vi "PXI4072 Set Refs.vi"(8 "error in (no error)":errorcluster, 11 "PXI4072 All UI Refs":T1) -> (0 "error out":errorcluster)   [LabVIEW 2026]
uses:
  App Types/References/PXI4072 All UI References.ctl
  App Types/References/PXI4072 Boolean UI References.ctl
  App Types/References/PXI4072 String UI References.ctl
  App Types/References/PXI4072 Numeric UI References.ctl
  App Types/References/PXI4072 Other UI Rerences.ctl
  Drivers/PXI4072/Types/PXI4072 Settings.ctl
  <instrlib>/niDMM/nidmm.llb/niDMM Function.ctl
  <instrlib>/niDMM/nidmm.llb/niDMM Resolution in Digits.ctl
  App Types/Globals/PXI4072 UI Global Refs.vi
  Drivers/PXI4072/PXI4072.lvlib
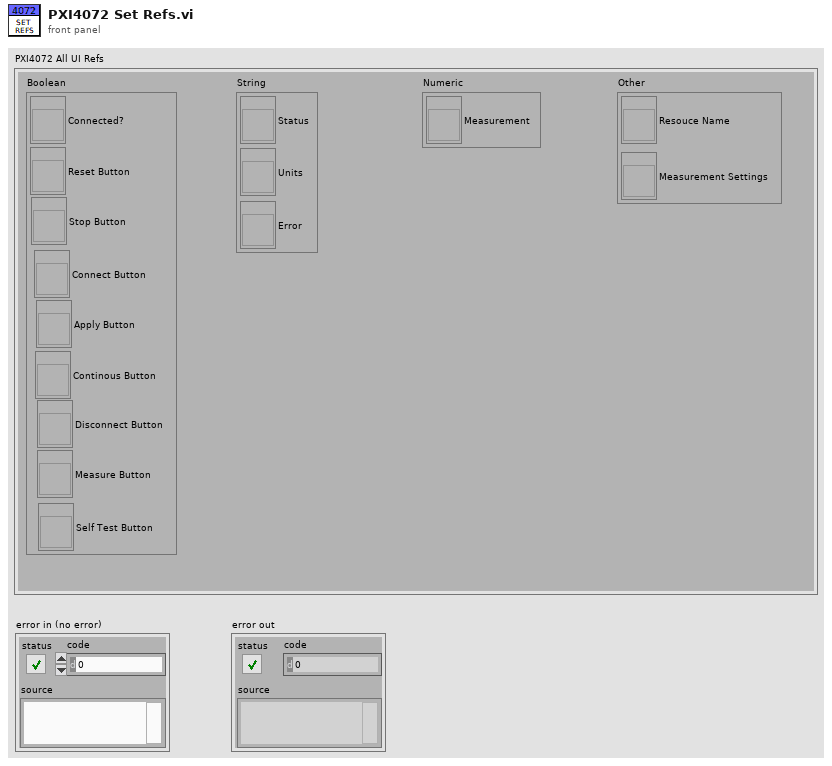
[diagram p1: front panel]
types:
  T1 = typedef "PXI4072 All UI References.ctl" = cluster{"Boolean":T2, "String":T3, "Numeric":T4, "Other":T5}
  T2 = typedef "PXI4072 Boolean UI References.ctl" = cluster{"Connected?":refnum<vi>, "Reset Button":refnum<vi>, "Connect Button":refnum<vi>, "Apply Button":refnum<vi>, "Disconnect Button":refnum<vi>, "Measure Button":refnum<vi>, "Self Test Button":refnum<vi>, "Continous Button":refnum<vi>, "Stop Button":refnum<vi>}
  T3 = typedef "PXI4072 String UI References.ctl" = cluster{"Status":refnum<vi>, "Units":refnum<vi>, "Error":refnum<vi>}
  T4 = typedef "PXI4072 Numeric UI References.ctl" = cluster{"Measurement":refnum<vi>}
  T5 = typedef "PXI4072 Other UI Rerences.ctl" = cluster{"Resouce Name":refnum<vi>, "Measurement Settings":refnum<vi>}
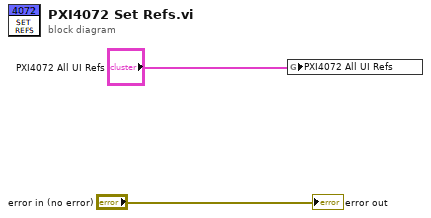
[diagram p0: block diagram]
diagram:
  n1 = global write "PXI4072 UI Global Refs.vi" "PXI4072 All UI Refs"("PXI4072 All UI Refs") -> ()
  "error out" <- "error in (no error)"
